vi "benchmark-TagDB2.vi"() -> (2 "read":dbl=2.8434400558471685e-05 format="%#_6f", 3 "write":dbl=2.78111743927002e-05 format="%#_6f")   [LabVIEW 2017]
uses:
  a6fc632b-2e92-436d-bf5a-00a40263cc33.vi
  5f513741-77c9-4122-96c3-2ffecd0507aa.vi
  TagDB/_Support/DataAccess/data-Write.vi
  TagDB/_Support/Error/_[error50000]Invalid DB REF.vi
  TagDB/_Support/DataAccess/TagDB Ref to DVR.vi
  TagDB/_Support/DataAccess/_NameCacher.vi
  TagDB/_Support/Error/_[error50002]Invalid DataType.vi
  TagDB/_Support/URL/TRIM-BOTH-SPACE.vi
  TagDB/_Support/DataAccess/_datatypeChecker.vi
  TagDB/_Support/Error/_Build Error Cluster.vi
  <vilib>/Utility/Data Type/Get Type Information.vi
  <vilib>/Utility/error.llb/Trim Whitespace.vi
  TagDB/TagDB.lvlib
panel:
  out "write 2":dbl=2.78111743927002e-05 caption="write" format="%#_6f"
  out "length":i32=1170
  out "outside":i32=499
  out "unit (s)":cluster{dbl[]}[](graph)=[{[4.010200500488281e-05, 2.005577087402344e-05, 3.0074119567871094e-05, 3.0078887939453124e-05, 3.0078887939453124e-05, 3.0078887939453124e-05, 2.0051002502441405e-05, 3.0078887939453124e-05, 3.0078887939453124e-05, 3.0078887939453124e-05, 3.0083656311035158e-05, 2.0847320556640624e-05, 2.9277801513671874e-05, 3.0078887939453124e-05, 3.0236244201660155e-05, 3.071784973144531e-05, 2.9430389404296874e-05, 2.002716064453125e-05, 2.9959678649902343e-05, 3.0078887939453124e-05, 3.0074119567871094e-05, 3.0231475830078124e-05, 2.0260810852050782e-05, 2.987384796142578e-05, 2.9926300048828124e-05, 3.0083656311035158e-05, 3.0069351196289064e-05, 3.0231475830078124e-05, 2.005577087402344e-05, 3.0074119567871094e-05, 2.9926300048828124e-05, 3.0078887939453124e-05, 3.0083656311035158e-05, 3.0078887939453124e-05, 2.0046234130859375e-05, 3.0088424682617188e-05, 3.0074119567871094e-05, 3.0078887939453124e-05, 3.0078887939453124e-05, 3.0078887939453124e-05, 2.0051002502441405e-05, 3.0078887939453124e-05, 3.0078887939453124e-05, 3.0078887939453124e-05, 3.0074119567871094e-05, 3.0078887939453124e-05, 2.005577087402344e-05, 3.0083656311035158e-05, 3.0078887939453124e-05, 3.0069351196289064e-05, 3.0083656311035158e-05, 3.0078887939453124e-05, 3.0078887939453124e-05, 2.0046234130859375e-05, 3.0083656311035158e-05, 3.0078887939453124e-05, 3.0078887939453124e-05, 3.0078887939453124e-05, 3.0083656311035158e-05, 2.0046234130859375e-05, 3.0078887939453124e-05, 3.0078887939453124e-05, 3.0083656311035158e-05, 3.0078887939453124e-05, 3.0069351196289064e-05, 2.006053924560547e-05, 3.0078887939453124e-05, 3.0078887939453124e-05, 3.0078887939453124e-05, 3.0074119567871094e-05, 2.005577087402344e-05, 3.0078887939453124e-05, 3.0078887939453124e-05, 3.0074119567871094e-05, 3.0078887939453124e-05, 3.0088424682617188e-05, 2.0046234130859375e-05, 3.0074119567871094e-05, 3.0078887939453124e-05, 3.0078887939453124e-05, 3.0083656311035158e-05, 3.0078887939453124e-05, 2.0046234130859375e-05, 3.0078887939453124e-05, 3.0083656311035158e-05, 3.0078887939453124e-05, 3.0078887939453124e-05, 3.0231475830078124e-05, 2.0051002502441405e-05, 2.9926300048828124e-05, 3.0078887939453124e-05, 3.0078887939453124e-05, 3.0074119567871094e-05, 2.005577087402344e-05, 3.0088424682617188e-05, 3.0074119567871094e-05, 3.0078887939453124e-05, 3.0069351196289064e-05, 2.005577087402344e-05, 3.0083656311035158e-05, 3.0078887939453124e-05, 3.0078887939453124e-05, 3.0074119567871094e-05, 3.0078887939453124e-05, 2.005577087402344e-05, 3.0069351196289064e-05, 3.0088424682617188e-05, 3.0074119567871094e-05, 3.0078887939453124e-05, 3.0078887939453124e-05, 3.0083656311035158e-05, 2.005577087402344e-05, 3.0069351196289064e-05, 3.0078887939453124e-05, 3.0083656311035158e-05, 3.0078887939453124e-05, 3.0078887939453124e-05, 2.0051002502441405e-05, 3.0078887939453124e-05, 3.0078887939453124e-05, 3.0078887939453124e-05, 3.0074119567871094e-05, 3.0078887939453124e-05, 2.005577087402344e-05, 3.0078887939453124e-05, 3.0083656311035158e-05, 3.0069351196289064e-05, 3.0078887939453124e-05, 3.024101257324219e-05, 2.0046234130859375e-05, 2.9931068420410158e-05, 3.0069351196289064e-05, 3.0088424682617188e-05, 3.0074119567871094e-05, 3.0231475830078124e-05, 3.0078887939453124e-05, 2.9931068420410158e-05, 3.0069351196289064e-05, 3.0078887939453124e-05, 2.005577087402344e-05, 2.0203590393066405e-05, 2.9931068420410158e-05, 3.0069351196289064e-05, 3.0083656311035158e-05, 3.0231475830078124e-05, 3.0078887939453124e-05, 2.005577087402344e-05, 2.9921531677246094e-05, 3.0078887939453124e-05, 3.0231475830078124e-05, 3.0078887939453124e-05, 3.0083656311035158e-05, 2.0046234130859375e-05, 2.9926300048828124e-05, 3.0078887939453124e-05, 3.0083656311035158e-05, 3.0069351196289064e-05, 2.02178955078125e-05, 3.0069351196289064e-05, 2.9931068420410158e-05, 3.0078887939453124e-05, 3.0074119567871094e-05, 3.0078887939453124e-05, 2.005577087402344e-05, 3.0078887939453124e-05, 3.0074119567871094e-05, 3.0078887939453124e-05, 3.0078887939453124e-05, 3.0078887939453124e-05, 3.0083656311035158e-05, 2.0046234130859375e-05, 3.0088424682617188e-05, 3.0069351196289064e-05, 3.0083656311035158e-05, 3.0078887939453124e-05, 3.0078887939453124e-05, 3.0074119567871094e-05, 2.005577087402344e-05, 3.0078887939453124e-05, 3.0078887939453124e-05, 3.0074119567871094e-05, 3.0078887939453124e-05, 3.0078887939453124e-05, 3.0078887939453124e-05, 2.005577087402344e-05, 3.0074119567871094e-05, 3.0078887939453124e-05, 3.0078887939453124e-05, 3.0083656311035158e-05, 3.0078887939453124e-05, 2.0046234130859375e-05, 3.0083656311035158e-05, 3.0078887939453124e-05, 3.0078887939453124e-05, 3.0078887939453124e-05, 3.0078887939453124e-05, 2.0051002502441405e-05, 3.0078887939453124e-05, 3.0231475830078124e-05, 3.0078887939453124e-05, 2.9931068420410158e-05, 3.0069351196289064e-05, 2.0847320556640624e-05, 2.944469451904297e-05, 3.0078887939453124e-05, 3.0069351196289064e-05, 2.9935836791992188e-05, 2.0203590393066405e-05, 3.071784973144531e-05, 2.9430389404296874e-05, 3.072261810302735e-05, 2.943992614746094e-05, 3.0078887939453124e-05, 2.005577087402344e-05, 3.0078887939453124e-05, 3.0074119567871094e-05, 3.0078887939453124e-05, 3.0078887939453124e-05, 3.0083656311035158e-05, 2.005577087402344e-05, 3.0069351196289064e-05, 3.072261810302735e-05, 2.943992614746094e-05, 3.0088424682617188e-05, 2.0046234130859375e-05, 3.0074119567871094e-05, 3.0078887939453124e-05, 3.0078887939453124e-05, 3.0078887939453124e-05, 3.0078887939453124e-05, 2.0051002502441405e-05, 3.0078887939453124e-05, 3.0078887939453124e-05, 3.0083656311035158e-05, 3.070831298828125e-05, 2.9449462890625e-05, 3.0078887939453124e-05, 2.0051002502441405e-05, 3.071784973144531e-05, 2.943992614746094e-05, 3.0074119567871094e-05, 3.0078887939453124e-05, 3.070354461669922e-05, 1.9431114196777344e-05, 3.0074119567871094e-05, 3.0078887939453124e-05, 3.0078887939453124e-05, 3.0112266540527343e-05, 3.005027770996094e-05, 2.005577087402344e-05, 3.0069351196289064e-05, 3.0078887939453124e-05, 3.0083656311035158e-05, 3.0078887939453124e-05, 3.0078887939453124e-05, 2.0051002502441405e-05, 3.0078887939453124e-05, 3.0078887939453124e-05, 3.0074119567871094e-05, 3.0083656311035158e-05, 3.0074119567871094e-05, 2.005577087402344e-05, 3.0078887939453124e-05, 3.0074119567871094e-05, 3.0078887939453124e-05, 3.0078887939453124e-05, 3.072261810302735e-05, 1.941680908203125e-05, 3.070831298828125e-05, 2.943992614746094e-05, 3.0083656311035158e-05, 3.0078887939453124e-05, 3.0078887939453124e-05, 2.0046234130859375e-05, 3.0083656311035158e-05, 3.0078887939453124e-05, 3.0078887939453124e-05, 3.0078887939453124e-05, 2.0051002502441405e-05, 3.071784973144531e-05, 2.943992614746094e-05, 3.0078887939453124e-05, 3.0083656311035158e-05, 3.0078887939453124e-05, 2.0046234130859375e-05, 3.0083656311035158e-05, 3.0078887939453124e-05, 3.0069351196289064e-05, 2.9935836791992188e-05, 3.0074119567871094e-05, 3.0078887939453124e-05, 2.0051002502441405e-05, 3.0231475830078124e-05, 3.0078887939453124e-05, 2.9926300048828124e-05, 3.0088424682617188e-05, 3.0074119567871094e-05, 3.0078887939453124e-05, 2.020835876464844e-05, 3.0069351196289064e-05, 2.9931068420410158e-05, 3.0078887939453124e-05, 3.0078887939453124e-05, 3.0074119567871094e-05, 3.0078887939453124e-05, 3.0078887939453124e-05, 2.0051002502441405e-05, 3.0078887939453124e-05, 3.0078887939453124e-05, 3.0078887939453124e-05, 3.0083656311035158e-05, 3.0078887939453124e-05, 3.0069351196289064e-05, 2.005577087402344e-05, 3.0083656311035158e-05, 3.0078887939453124e-05, 3.0078887939453124e-05, 3.0074119567871094e-05, 3.0078887939453124e-05, 2.005577087402344e-05, 3.0078887939453124e-05, 3.0074119567871094e-05, 3.0078887939453124e-05, 3.0078887939453124e-05, 3.0078887939453124e-05, 2.0051002502441405e-05, 3.0078887939453124e-05, 3.024101257324219e-05, 3.0069351196289064e-05, 2.9931068420410158e-05, 2.0046234130859375e-05, 3.024101257324219e-05, 3.0112266540527343e-05, 2.9888153076171875e-05, 3.0112266540527343e-05, 3.0045509338378905e-05, 3.0078887939453124e-05, 2.0051002502441405e-05, 3.0078887939453124e-05, 3.0231475830078124e-05, 3.0078887939453124e-05, 2.9931068420410158e-05, 3.0069351196289064e-05, 2.0847320556640624e-05, 2.943992614746094e-05, 3.072261810302735e-05, 2.9430389404296874e-05, 3.0083656311035158e-05, 3.0078887939453124e-05, 2.005577087402344e-05, 3.0078887939453124e-05, 3.0074119567871094e-05, 2.9935836791992188e-05, 3.0221939086914064e-05, 3.0078887939453124e-05, 2.005577087402344e-05, 3.071308135986328e-05, 2.943992614746094e-05, 3.0112266540527343e-05, 3.005027770996094e-05, 3.071784973144531e-05, 2.943992614746094e-05, 2.0046234130859375e-05, 3.0083656311035158e-05, 2.9926300048828124e-05, 3.0231475830078124e-05, 3.0078887939453124e-05, 2.0051002502441405e-05, 3.0078887939453124e-05, 3.071784973144531e-05, 2.943992614746094e-05, 3.0074119567871094e-05, 3.0078887939453124e-05, 2.0694732666015624e-05, 2.9435157775878905e-05, 3.0078887939453124e-05, 3.0088424682617188e-05, 3.0074119567871094e-05, 3.0078887939453124e-05, 2.0046234130859375e-05, 3.0078887939453124e-05, 3.0083656311035158e-05, 3.0078887939453124e-05, 3.0088424682617188e-05, 2.0046234130859375e-05, 3.0074119567871094e-05, 3.0078887939453124e-05, 3.0078887939453124e-05, 3.0078887939453124e-05, 3.0083656311035158e-05, 2.0046234130859375e-05, 3.0078887939453124e-05, 3.0078887939453124e-05, 3.0074119567871094e-05, 3.0078887939453124e-05, 3.0078887939453124e-05, 2.005577087402344e-05, 3.0083656311035158e-05, 3.0078887939453124e-05, 3.0088424682617188e-05, 3.006458282470703e-05, 3.0078887939453124e-05, 2.005577087402344e-05, 3.0074119567871094e-05, 3.0078887939453124e-05, 3.0078887939453124e-05, 3.0078887939453124e-05, 3.0083656311035158e-05, 3.0078887939453124e-05, 2.0046234130859375e-05, 3.0078887939453124e-05, 3.0083656311035158e-05, 3.0078887939453124e-05, 3.0078887939453124e-05, 3.0074119567871094e-05, 3.0078887939453124e-05, 2.0694732666015624e-05, 2.943992614746094e-05, 3.0078887939453124e-05, 3.0083656311035158e-05, 3.070831298828125e-05, 2.943992614746094e-05, 2.005577087402344e-05, 2.9931068420410158e-05, 3.0069351196289064e-05, 3.0231475830078124e-05, 3.0083656311035158e-05, 3.009319305419922e-05, 3.005504608154297e-05, 1.99127197265625e-05, 3.0226707458496094e-05, 3.0078887939453124e-05, 3.0078887939453124e-05, 3.072261810302735e-05, 2.928733825683594e-05, 2.0046234130859375e-05, 3.0078887939453124e-05, 3.0236244201660155e-05, 3.0069351196289064e-05, 3.025054931640625e-05, 2.9764175415039063e-05, 2.0051002502441405e-05, 3.0069351196289064e-05, 3.0088424682617188e-05, 3.0226707458496094e-05, 3.0078887939453124e-05, 2.9926300048828124e-05, 2.0051002502441405e-05, 3.0078887939453124e-05, 3.0078887939453124e-05, 3.0078887939453124e-05, 3.0231475830078124e-05, 2.9931068420410158e-05, 2.0046234130859375e-05, 3.0078887939453124e-05, 3.0083656311035158e-05, 3.0231475830078124e-05, 2.9926300048828124e-05, 2.0046234130859375e-05, 3.0083656311035158e-05, 3.0078887939453124e-05, 3.0078887939453124e-05, 3.0231475830078124e-05, 2.9921531677246094e-05, 3.0088424682617188e-05, 2.0046234130859375e-05, 3.0074119567871094e-05, 3.0078887939453124e-05, 3.0078887939453124e-05, 3.0078887939453124e-05, 3.0083656311035158e-05, 2.005577087402344e-05, 3.0069351196289064e-05, 3.0083656311035158e-05, 3.0078887939453124e-05, 3.0078887939453124e-05, 3.0078887939453124e-05, 2.0051002502441405e-05, 3.0078887939453124e-05, 3.0231475830078124e-05, 3.0078887939453124e-05, 2.9931068420410158e-05, 3.0078887939453124e-05, 2.0046234130859375e-05, 3.0078887939453124e-05, 3.0231475830078124e-05, 3.0083656311035158e-05, 2.9926300048828124e-05, 3.0074119567871094e-05, 2.0847320556640624e-05, 2.9430389404296874e-05, 2.9926300048828124e-05, 3.0083656311035158e-05, 3.0088424682617188e-05, 3.0069351196289064e-05, 2.0051002502441405e-05, 3.0078887939453124e-05, 3.0078887939453124e-05, 3.0078887939453124e-05, 3.0078887939453124e-05]}, ...(2 in all)]
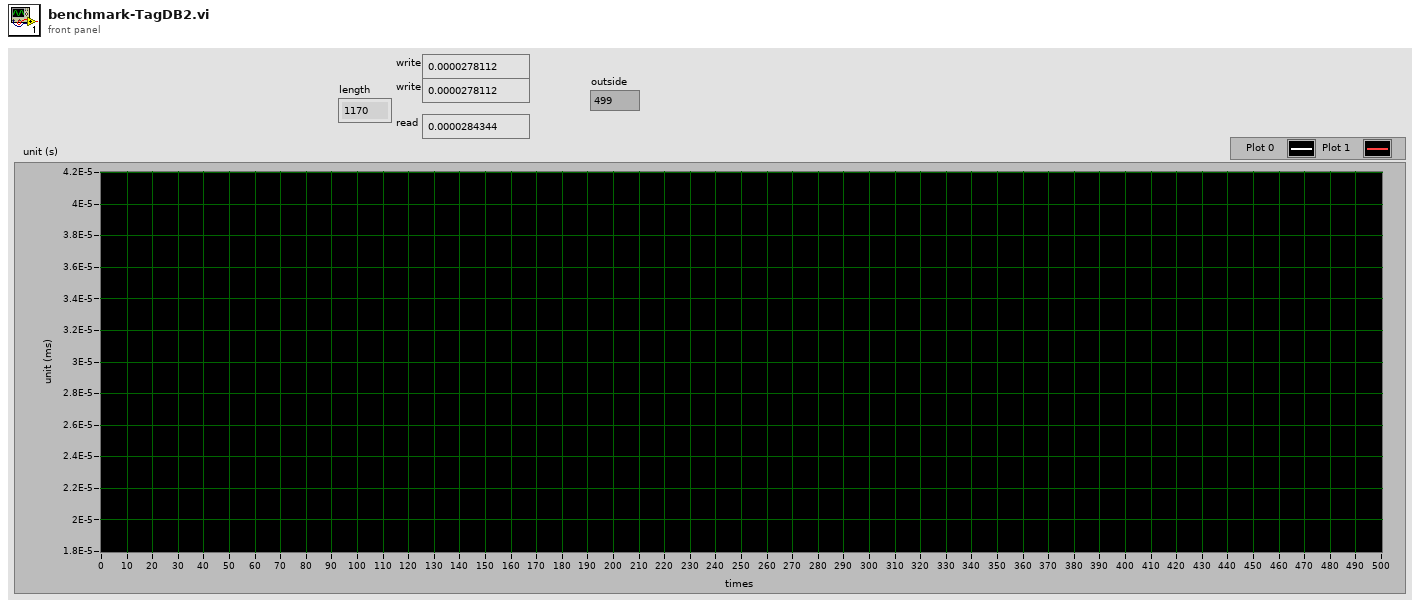
[diagram p1: front panel]
types:
  T1 = cluster{"error constant":errorcluster, "error constant 2":errorcluster, "error constant 3":errorcluster, "error constant 4":errorcluster, "error constant 5":errorcluster, "error constant 6":errorcluster, "error constant 7":errorcluster, "error constant 8":errorcluster, "error constant 9":errorcluster, "error constant 10":errorcluster, "error constant 11":errorcluster, "error constant 12":errorcluster, "error constant 13":errorcluster, "error constant 14":errorcluster, "error constant 15":errorcluster, "error constant 16":errorcluster, "error constant 17":errorcluster, "error constant 18":errorcluster, "error constant 19":errorcluster, "error constant 20":errorcluster, "error constant 21":errorcluster, "error constant 22":errorcluster, "error constant 23":errorcluster, "error constant 24":errorcluster, "error constant 25":errorcluster, "error constant 26":errorcluster, "error constant 27":errorcluster, "error constant 28":errorcluster, "error constant 29":errorcluster, "error constant 30":errorcluster, "error constant 31":errorcluster, "error constant 32":errorcluster, "error constant 33":errorcluster, "error constant 34":errorcluster, "error constant 35":errorcluster, "error constant 36":errorcluster, "error constant 37":errorcluster, "error constant 38":errorcluster, "error constant 39":errorcluster, "error constant 40":errorcluster, "error constant 41":errorcluster, "error constant 42":errorcluster, "error constant 43":errorcluster, "error constant 44":errorcluster, "error constant 45":errorcluster, "error constant 46":errorcluster, "error constant 47":errorcluster, "error constant 48":errorcluster, "error constant 49":errorcluster, "error constant 50":errorcluster, "error constant 51":errorcluster, "error constant 52":errorcluster, "error constant 53":errorcluster, "error constant 54":errorcluster, "error constant 55":errorcluster, "error constant 56":errorcluster, "error constant 57":errorcluster, "error constant 58":errorcluster, "error constant 59":errorcluster, "error constant 60":errorcluster, "error constant 61":errorcluster, "error constant 62":errorcluster, "error constant 63":errorcluster, "error constant 64":errorcluster, "error constant 65":errorcluster, cluster{"error constant":errorcluster, "error constant 2":errorcluster, "error constant 3":errorcluster, "error constant 4":errorcluster, "error constant 5":errorcluster, "error constant 6":errorcluster, "error constant 7":errorcluster, "error constant 8":errorcluster, "error constant 9":errorcluster, "error constant 10":errorcluster, "error constant 11":errorcluster, "error constant 12":errorcluster, "error constant 13":errorcluster, "error constant 14":errorcluster, "error constant 15":errorcluster, "error constant 16":errorcluster, "error constant 17":errorcluster, "error constant 18":errorcluster, "error constant 19":errorcluster, "error constant 20":errorcluster, "error constant 21":errorcluster, "error constant 22":errorcluster, "error constant 23":errorcluster, "error constant 24":errorcluster, "error constant 25":errorcluster, "error constant 26":errorcluster, "error constant 27":errorcluster, "error constant 28":errorcluster, "error constant 29":errorcluster, "error constant 30":errorcluster, "error constant 31":errorcluster, "error constant 32":errorcluster, "error constant 33":errorcluster, "error constant 34":errorcluster, "error constant 35":errorcluster, "error constant 36":errorcluster, "error constant 37":errorcluster, "error constant 38":errorcluster, "error constant 39":errorcluster, "error constant 40":errorcluster, "error constant 41":errorcluster, "error constant 42":errorcluster, "error constant 43":errorcluster, "error constant 44":errorcluster, "error constant 45":errorcluster, "error constant 46":errorcluster, "error constant 47":errorcluster, "error constant 48":errorcluster, "error constant 49":errorcluster, "error constant 50":errorcluster, "error constant 51":errorcluster, "error constant 52":errorcluster, "error constant 53":errorcluster, "error constant 54":errorcluster, "error constant 55":errorcluster, "error constant 56":errorcluster, "error constant 57":errorcluster, "error constant 58":errorcluster, "error constant 59":errorcluster, "error constant 60":errorcluster, "error constant 61":errorcluster, "error constant 62":errorcluster, "error constant 63":errorcluster, "error constant 64":errorcluster, "error constant 65":errorcluster}}
  T2 = typedef "TagDB.lvlib/TagDB.ctl" = refnum<k1>
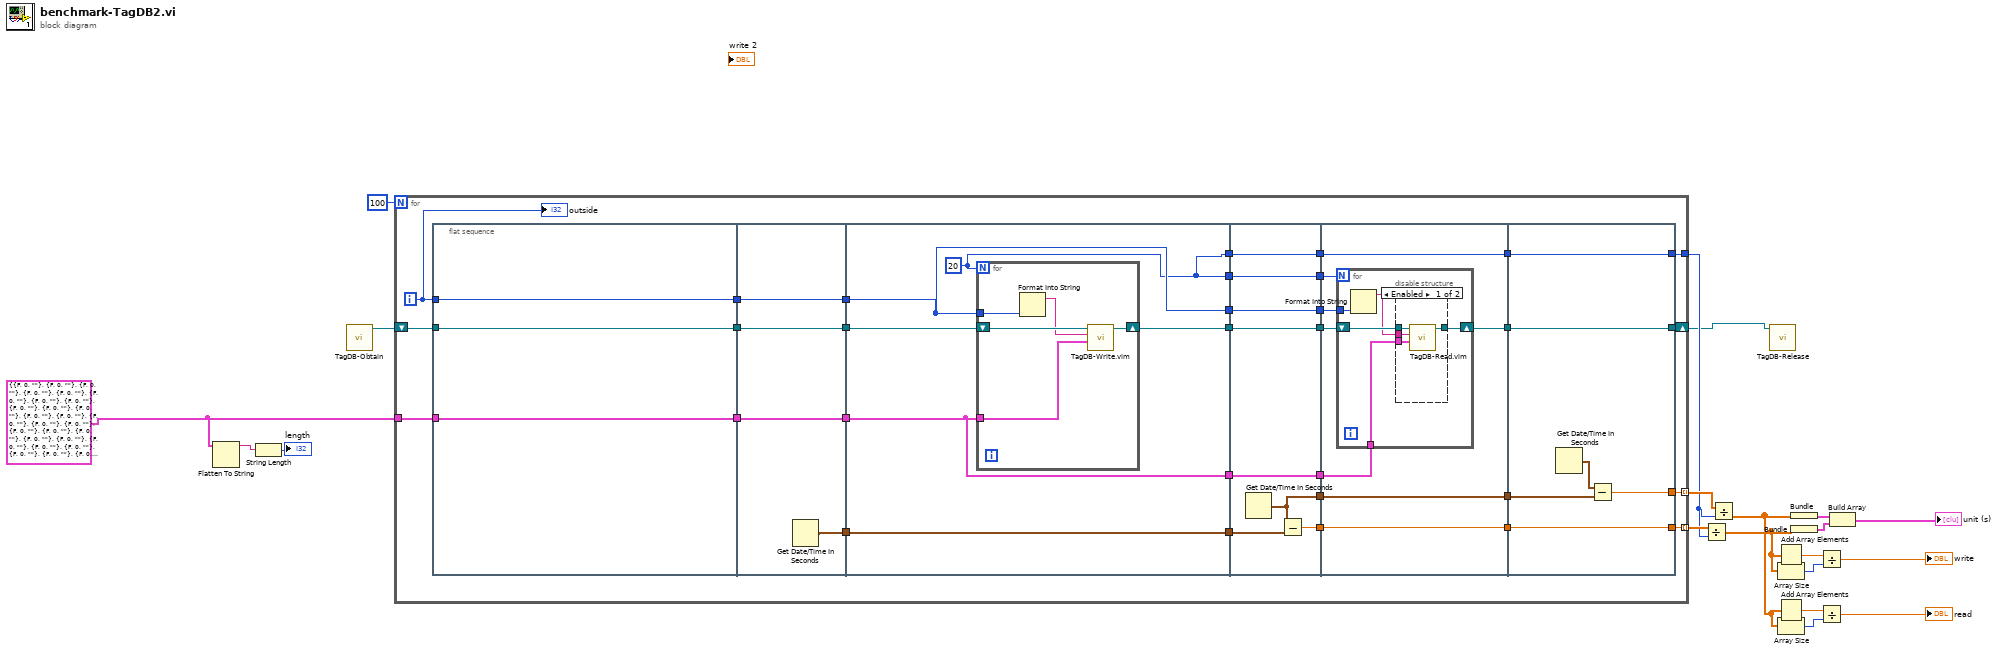
[diagram p0: block diagram]
diagram:
  w17 = T1 {"error constant"={"status"=FALSE, "code"=0, "source"=""}, "error constant 2"={"status"=FALSE, "code"=0, "source"=""}, "error constant 3"={"status"=FALSE, "code"=0, "source"=""}, "error constant 4"={"status"=FALSE, "code"=0, "source"=""}, "error constant 5"={"status"=FALSE, "code"=0, "source"=""}, "error constant 6"={"status"=FALSE, "code"=0, "source"=""}, "error constant 7"={"status"=FALSE, "code"=0, "source"=""}, "error constant 8"={"status"=FALSE, "code"=0, "source"=""}, "error constant 9"={"status"=FALSE, "code"=0, "source"=""}, "error constant 10"={"status"=FALSE, "code"=0, "source"=""}, "error constant 11"={"status"=FALSE, "code"=0, "source"=""}, "error constant 12"={"status"=FALSE, "code"=0, "source"=""}, "error constant 13"={"status"=FALSE, "code"=0, "source"=""}, "error constant 14"={"status"=FALSE, "code"=0, "source"=""}, "error constant 15"={"status"=FALSE, "code"=0, "source"=""}, "error constant 16"={"status"=FALSE, "code"=0, "source"=""}, "error constant 17"={"status"=FALSE, "code"=0, "source"=""}, "error constant 18"={"status"=FALSE, "code"=0, "source"=""}, "error constant 19"={"status"=FALSE, "code"=0, "source"=""}, "error constant 20"={"status"=FALSE, "code"=0, "source"=""}, "error constant 21"={"status"=FALSE, "code"=0, "source"=""}, "error constant 22"={"status"=FALSE, "code"=0, "source"=""}, "error constant 23"={"status"=FALSE, "code"=0, "source"=""}, "error constant 24"={"status"=FALSE, "code"=0, "source"=""}, "error constant 25"={"status"=FALSE, "code"=0, "source"=""}, "error constant 26"={"status"=FALSE, "code"=0, "source"=""}, "error constant 27"={"status"=FALSE, "code"=0, "source"=""}, "error constant 28"={"status"=FALSE, "code"=0, "source"=""}, "error constant 29"={"status"=FALSE, "code"=0, "source"=""}, "error constant 30"={"status"=FALSE, "code"=0, "source"=""}, "error constant 31"={"status"=FALSE, "code"=0, "source"=""}, "error constant 32"={"status"=FALSE, "code"=0, "source"=""}, "error constant 33"={"status"=FALSE, "code"=0, "source"=""}, "error constant 34"={"status"=FALSE, "code"=0, "source"=""}, "error constant 35"={"status"=FALSE, "code"=0, "source"=""}, "error constant 36"={"status"=FALSE, "code"=0, "source"=""}, "error constant 37"={"status"=FALSE, "code"=0, "source"=""}, "error constant 38"={"status"=FALSE, "code"=0, "source"=""}, "error constant 39"={"status"=FALSE, "code"=0, "source"=""}, "error constant 40"={"status"=FALSE, "code"=0, "source"=""}, "error constant 41"={"status"=FALSE, "code"=0, "source"=""}, "error constant 42"={"status"=FALSE, "code"=0, "source"=""}, "error constant 43"={"status"=FALSE, "code"=0, "source"=""}, "error constant 44"={"status"=FALSE, "code"=0, "source"=""}, "error constant 45"={"status"=FALSE, "code"=0, "source"=""}, "error constant 46"={"status"=FALSE, "code"=0, "source"=""}, "error constant 47"={"status"=FALSE, "code"=0, "source"=""}, "error constant 48"={"status"=FALSE, "code"=0, "source"=""}, "error constant 49"={"status"=FALSE, "code"=0, "source"=""}, "error constant 50"={"status"=FALSE, "code"=0, "source"=""}, "error constant 51"={"status"=FALSE, "code"=0, "source"=""}, "error constant 52"={"status"=FALSE, "code"=0, "source"=""}, "error constant 53"={"status"=FALSE, "code"=0, "source"=""}, "error constant 54"={"status"=FALSE, "code"=0, "source"=""}, "error constant 55"={"status"=FALSE, "code"=0, "source"=""}, "error constant 56"={"status"=FALSE, "code"=0, "source"=""}, "error constant 57"={"status"=FALSE, "code"=0, "source"=""}, "error constant 58"={"status"=FALSE, "code"=0, "source"=""}, "error constant 59"={"status"=FALSE, "code"=0, "source"=""}, "error constant 60"={"status"=FALSE, "code"=0, "source"=""}, "error constant 61"={"status"=FALSE, "code"=0, "source"=""}, "error constant 62"={"status"=FALSE, "code"=0, "source"=""}, "error constant 63"={"status"=FALSE, "code"=0, "source"=""}, "error constant 64"={"status"=FALSE, "code"=0, "source"=""}, "error constant 65"={"status"=FALSE, "code"=0, "source"=""}, {"error constant"={"status"=FALSE, "code"=0, "source"=""}, "error constant 2"={"status"=FALSE, "code"=0, "source"=""}, "error constant 3"={"status"=FALSE, "code"=0, "source"=""}, "error constant 4"={"status"=FALSE, "code"=0, "source"=""}, "error constant 5"={"status"=FALSE, "code"=0, "source"=""}, "error constant 6"={"status"=FALSE, "code"=0, "source"=""}, "error constant 7"={"status"=FALSE, "code"=0, "source"=""}, "error constant 8"={"status"=FALSE, "code"=0, "source"=""}, "error constant 9"={"status"=FALSE, "code"=0, "source"=""}, "error constant 10"={"status"=FALSE, "code"=0, "source"=""}, "error constant 11"={"status"=FALSE, "code"=0, "source"=""}, "error constant 12"={"status"=FALSE, "code"=0, "source"=""}, "error constant 13"={"status"=FALSE, "code"=0, "source"=""}, "error constant 14"={"status"=FALSE, "code"=0, "source"=""}, "error constant 15"={"status"=FALSE, "code"=0, "source"=""}, "error constant 16"={"status"=FALSE, "code"=0, "source"=""}, "error constant 17"={"status"=FALSE, "code"=0, "source"=""}, "error constant 18"={"status"=FALSE, "code"=0, "source"=""}, "error constant 19"={"status"=FALSE, "code"=0, "source"=""}, "error constant 20"={"status"=FALSE, "code"=0, "source"=""}, "error constant 21"={"status"=FALSE, "code"=0, "source"=""}, "error constant 22"={"status"=FALSE, "code"=0, "source"=""}, "error constant 23"={"status"=FALSE, "code"=0, "source"=""}, "error constant 24"={"status"=FALSE, "code"=0, "source"=""}, "error constant 25"={"status"=FALSE, "code"=0, "source"=""}, "error constant 26"={"status"=FALSE, "code"=0, "source"=""}, "error constant 27"={"status"=FALSE, "code"=0, "source"=""}, "error constant 28"={"status"=FALSE, "code"=0, "source"=""}, "error constant 29"={"status"=FALSE, "code"=0, "source"=""}, "error constant 30"={"status"=FALSE, "code"=0, "source"=""}, "error constant 31"={"status"=FALSE, "code"=0, "source"=""}, "error constant 32"={"status"=FALSE, "code"=0, "source"=""}, "error constant 33"={"status"=FALSE, "code"=0, "source"=""}, "error constant 34"={"status"=FALSE, "code"=0, "source"=""}, "error constant 35"={"status"=FALSE, "code"=0, "source"=""}, "error constant 36"={"status"=FALSE, "code"=0, "source"=""}, "error constant 37"={"status"=FALSE, "code"=0, "source"=""}, "error constant 38"={"status"=FALSE, "code"=0, "source"=""}, "error constant 39"={"status"=FALSE, "code"=0, "source"=""}, "error constant 40"={"status"=FALSE, "code"=0, "source"=""}, "error constant 41"={"status"=FALSE, "code"=0, "source"=""}, "error constant 42"={"status"=FALSE, "code"=0, "source"=""}, "error constant 43"={"status"=FALSE, "code"=0, "source"=""}, "error constant 44"={"status"=FALSE, "code"=0, "source"=""}, "error constant 45"={"status"=FALSE, "code"=0, "source"=""}, "error constant 46"={"status"=FALSE, "code"=0, "source"=""}, "error constant 47"={"status"=FALSE, "code"=0, "source"=""}, "error constant 48"={"status"=FALSE, "code"=0, "source"=""}, "error constant 49"={"status"=FALSE, "code"=0, "source"=""}, "error constant 50"={"status"=FALSE, "code"=0, "source"=""}, "error constant 51"={"status"=FALSE, "code"=0, "source"=""}, "error constant 52"={"status"=FALSE, "code"=0, "source"=""}, "error constant 53"={"status"=FALSE, "code"=0, "source"=""}, "error constant 54"={"status"=FALSE, "code"=0, "source"=""}, "error constant 55"={"status"=FALSE, "code"=0, "source"=""}, "error constant 56"={"status"=FALSE, "code"=0, "source"=""}, "error constant 57"={"status"=FALSE, "code"=0, "source"=""}, "error constant 58"={"status"=FALSE, "code"=0, "source"=""}, "error constant 59"={"status"=FALSE, "code"=0, "source"=""}, "error constant 60"={"status"=FALSE, "code"=0, "source"=""}, "error constant 61"={"status"=FALSE, "code"=0, "source"=""}, "error constant 62"={"status"=FALSE, "code"=0, "source"=""}, "error constant 63"={"status"=FALSE, "code"=0, "source"=""}, "error constant 64"={"status"=FALSE, "code"=0, "source"=""}, "error constant 65"={"status"=FALSE, "code"=0, "source"=""}}}
  n1 = Flatten To String(anything=w17) -> (data string=w16:string)  [unwired: 3 in, 2 out]
  n2 = String Length(string=w16) -> (length=→"length":i32)
  n3 = call "TagDB-Obtain.vi"() -> ("TagDB"=w2:T2)  [unwired: 5 in, 2 out]
  n4 = for {
    N: 100 -> [_]
    tunnel: [w49] -> w20 mode=indexing
    tunnel: [w48] -> w3
    tunnel: w17 -> [w35]
    shift-right: [w33] -> w1
    shift-left: w2 -> [w34]
    tunnel: [w28] -> w4 mode=indexing
    i -> [w46]
    n5 = flat-sequence {
      tunnel: w46 -> [w54]
      tunnel: [w52] -> w40
      tunnel: [w53] -> w38
      tunnel: [w54] -> w37
      tunnel: w35 -> [w53]
      tunnel: w34 -> [w52]
      tunnel: [w58] -> w51
      tunnel: [w57] -> w41
      tunnel: w40 -> [w57]
      tunnel: [w56] -> w39
      tunnel: w38 -> [w56]
      tunnel: w37 -> [w55]
      tunnel: [w55] -> w36
      tunnel: w51 -> [w64]
      tunnel: [w64] -> w50
      tunnel: [w60] -> w47
      tunnel: [w62] -> w42
      tunnel: w41 -> [w63]
      tunnel: w39 -> [w59]
      tunnel: w36 -> [w61]
      tunnel: [w60] -> w26
      tunnel: [w61] -> w23
      tunnel: [w59] -> w22
      tunnel: w50 -> [w74]
      tunnel: w47 -> [w76]
      tunnel: [w77] -> w45
      tunnel: [w76] -> w44
      tunnel: [w75] -> w43
      tunnel: w42 -> [w75]
      tunnel: [w70] -> w30
      tunnel: w26 -> [w73]
      tunnel: [w73] -> w25
      tunnel: [w72] -> w24
      tunnel: w23 -> [w72]
      tunnel: w22 -> [w71]
      tunnel: [w71] -> w21
      tunnel: w45 -> [w85]
      tunnel: w44 -> [w84]
      tunnel: w43 -> [w82]
      tunnel: [w85] -> w32
      tunnel: [w84] -> w31
      tunnel: w30 -> [w83]
      tunnel: [w83] -> w29
      tunnel: [w81] -> w27
      tunnel: w25 -> [w80]
      tunnel: w24 -> [w79]
      tunnel: w21 -> [w78]
      tunnel: [w99] -> w33
      tunnel: [w100] -> w48
      tunnel: [w101] -> w49
      tunnel: w32 -> [w101]
      tunnel: w31 -> [w100]
      tunnel: w29 -> [w97]
      tunnel: [w96] -> w28
      tunnel: w27 -> [w99]
      frame #0 {
      }
      frame #1 {
        n6 = Get Date/Time In Seconds() -> (seconds since 1Jan1904=w58:timestamp)
      }
      frame #2 {
        w60 = 20
        n7 = for {
          N: w60 -> [_]
          tunnel: w59 -> [w66]
          tunnel: w61 -> [w69]
          shift-right: [w67] -> w62
          shift-left: w63 -> [w68]
          n8 = Format Into String(w69) -> (resulting string=w65:string)  [unwired: 3 in, 1 out]
          n9 = call "TagDB-Write.vim"("Value"=w66, "name"=w65, "TagDB"=w68) -> ("TagDB(dup)"=w67:T2)  [unwired: 6 in, 2 out]
        }
      }
      frame #3 {
        n10 = Get Date/Time In Seconds() -> (seconds since 1Jan1904=w70:timestamp)
        n11 = Subtract(x=w70, y=w74) -> (x-y=w77:dbl)
      }
      frame #4 {
        n12 = for {
          N: w80 -> [_]
          shift-right: [w89] -> w81
          shift-left: w82 -> [w88]
          tunnel: w79 -> [w90]
          tunnel: w78 -> [w86]
          n13 = Format Into String(w90) -> (resulting string=w87:string)  [unwired: 3 in, 1 out]
          n14 = disable-structure shown="Enabled" {
            disable-tunnel: [w94 w95] -> w89
            disable-tunnel: w88 -> [w93 w95]
            disable-tunnel: w87 -> [w92 _]
            disable-tunnel: w86 -> [w91 _]
            frame Enabled {
              n15 = call "TagDB-Read.vim"("Type(empty to read as variant)"=w91, "name"=w92, "TagDB"=w93) -> ("TagDB(dup)"=w94:T2)  [unwired: 3 in, 5 out]
            }
            frame Disabled {
            }
          }
        }
      }
      frame #5 {
        n16 = Get Date/Time In Seconds() -> (seconds since 1Jan1904=w98:timestamp)
        n17 = Subtract(x=w98, y=w97) -> (x-y=w96:dbl)
      }
    }
    "outside" <- w46
  }
  n18 = Divide(x=w20, y=w3) -> (x/y=w12:dbl[])
  n19 = Divide(x=w4, y=w3) -> (x/y=w5:dbl[])
  n20 = call "TagDB-Release.vi"("TagDB"=w1) -> ()  [unwired: 10 in, 1 out]
  n21 = Add Array Elements(numeric array=w12) -> (sum=w14:dbl)
  n22 = Array Size(array=w12) -> (size(s)=w13:i32)
  n23 = Add Array Elements(numeric array=w5) -> (sum=w7:dbl)
  n24 = Array Size(array=w5) -> (size(s)=w8:i32)
  n25 = Bundle(w5) -> (w11:cluster{dbl[]})  [unwired: 1 in]
  n26 = Bundle(w12) -> (w10:cluster{dbl[]})  [unwired: 1 in]
  n27 = Divide(x=w14, y=w13) -> (x/y=→"write":dbl)
  n28 = Divide(x=w7, y=w8) -> (x/y=→"read":dbl)
  n29 = Build Array(w11, w10) -> (→"unit (s)":cluster{dbl[]}[])
